vi "4.7.vi"() -> ()   [LabVIEW 2019]
panel:
  in  "a":dbl
  in  "f":dbl
  out "Waveform Graph":dynamicdata(graph)
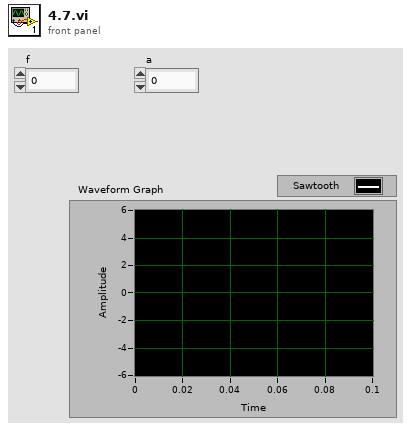
[diagram p1: front panel]
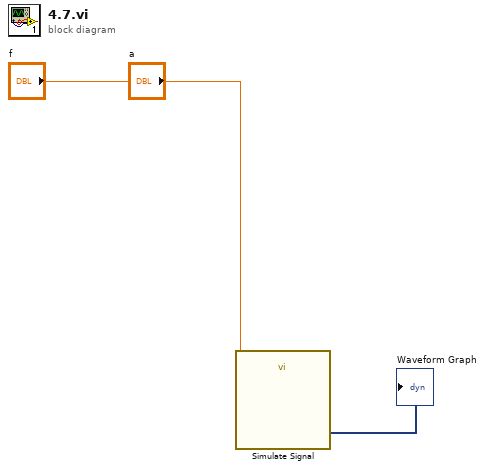
[diagram p0: block diagram]
diagram:
  n1 = call "Simulate Signal"("Frequency"="f", "Amplitude"="a") -> ("Sawtooth"=→"Waveform Graph":dynamicdata)  [unwired: 12 in, 1 out]
